vi "BIO_find_type.vi"(8 "error in (no error)":errorcluster, 11 "BIO in":refnum<class "BIO.lvclass">) -> (0 "error out":errorcluster, 2 "Found BIO":refnum<class "BIO.lvclass">, 3 "BIO out":refnum<class "BIO.lvclass">)   [LabVIEW 2013, in "SSL_Lib.lvlib" / "BIO.lvclass"]
uses:
  BIO.lvclass
  BIO Type.ctl
  SSL-Lib/SSL-Lib.lvclass/SSL-Lib.ctl
  BIO.lvclass/BIO.ctl
  SSL-Lib/Read Crypto Library Path.vi
  Read Handle.vi
  Write Handle.vi
  SSL-Lib/SSL-Lib.lvclass
panel:
  in  "BIO Type":T1 items=["BIO_TYPE_SOCKET"=1285]
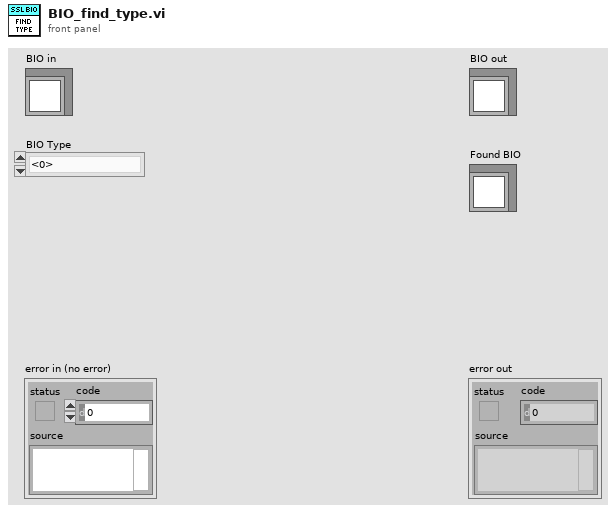
[diagram p1: front panel]
types:
  T1 = typedef "SSL_Lib.lvlib/BIO.lvclass/BIO Type.ctl" = i32
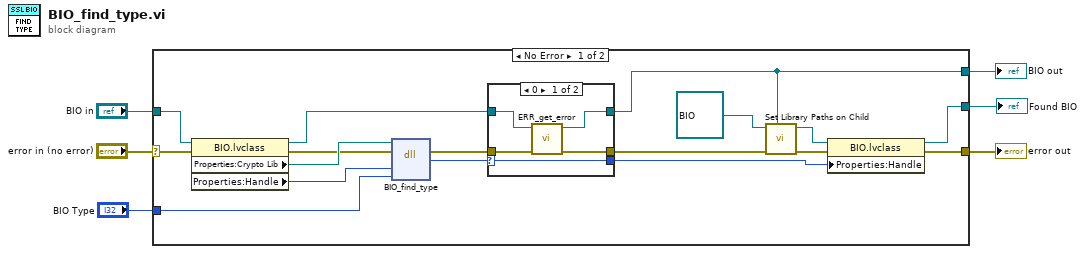
[diagram p0: block diagram]
diagram:
  n1 = case shown="No Error" "error in (no error)" {
    selector: "error in (no error)" -> [w22 w33]
    tunnel: [w11 w33] -> w5
    tunnel: [w13 w32] -> w3
    tunnel: "BIO in" -> [w23 w32]
    tunnel: [w10 _] -> w2
    tunnel: "BIO Type" -> [w7 _]
    frame No Error {
      n2 = property class="BIO.lvclass"(reference=w23, error in=w22) -> (reference out=w16:refnum<class "BIO.lvclass">, error out=w19:errorcluster, "Properties:Crypto Lib"=w21:path, "Properties:Handle"=w20:u64)
      n3 = dll-call lib="C:/Program Files (x86)/National Instruments/Shared/nissl/NIlibeay32.dll" fn="BIO_find_type"(path in=w21, error in=w19, "BIO"=w20, "type"=w7) -> (error out=w17:errorcluster, "return type"=w18:u64)  [unwired: 3 in, 1 out]
      n4 = case shown="0" w18 {
        selector: w18 -> [w24 w29]
        tunnel: w17 -> [w28 w31]
        tunnel: [w25 w31] -> w15
        tunnel: w16 -> [w27 w30]
        tunnel: [w26 w30] -> w13
        tunnel: [w24 w29] -> w8
        frame 0 {
          n5 = call "ERR_get_error.vi"("error in (no error)"=w28, "SSL-Lib in"=w27) -> ("error out"=w25:errorcluster, "SSL-Lib out"=w26:refnum<class "BIO.lvclass">)  [unwired: 8 in]
        }
        frame Default {
        }
      }
      n6 = call-dynamic "Set Library Paths on Child.vi"(7:"SSL-Lib in"=w13, "error in (no error)"=w15, 11:"SSL-Lib in"=refnum<class "BIO.lvclass"> refnum ("Popped BIO")) -> ("error out"=w14:errorcluster, "SSL-Lib out"=w12:refnum<class "BIO.lvclass">)  [unwired: 7 in]
      n7 = property class="BIO.lvclass"(reference=w12, error in=w14, "Properties:Handle"=w8) -> (reference out=w10:refnum<class "BIO.lvclass">, error out=w11:errorcluster)
    }
    frame Error {
    }
  }
  "error out" <- w5
  "BIO out" <- w3
  "Found BIO" <- w2
